vi "Write Colors.vi"(5 "Colors":T1, 9 "Decoration in":refnum<class "Decoration.lvclass">) -> (3 "Decoration out":refnum<class "Decoration.lvclass">)   [LabVIEW 2014, in "Decoration.lvclass"]
uses:
  Decoration.lvclass
  <vilib>/Utility/miscctls.llb/LVForegroundBackgroundColorsTypeDef.ctl
  Decoration.lvclass/Decoration.ctl
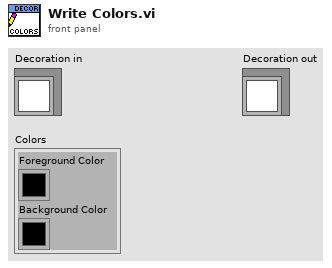
[diagram p1: front panel]
types:
  T1 = typedef "LVForegroundBackgroundColorsTypeDef.ctl" = cluster{"Foreground Color":u32, "Background Color":u32}
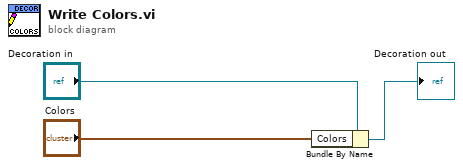
[diagram p0: block diagram]
diagram:
  n1 = Bundle By Name(cluster="Decoration in", "Colors"="Colors") -> (→"Decoration out":refnum<class "Decoration.lvclass">)
